vi "phasePlotWrap.vi"(6 "Sampling info":cluster{"Fs":dbl, "#s":dbl}={"Fs"=10000.0, "#s"=1000.0} {"Fs" format="%.2p"}, 8 "Phase unit":u16(ring) items=["Degree", "Radian"], 9 "Phase":dbl, 10 "Nomial Frequency":dbl, 11 "Frequency":dbl) -> (1 "yScaleMin":dbl, 2 "yScaleMax":dbl, 3 "Phase waveform":waveform(dbl)(graph))   [LabVIEW 2025]
uses:
  <vilib>/measure/NI_MAPro.lvlib
  <vilib>/measure/maresamp.llb/Align 1 + N Waveforms (continuous).vi
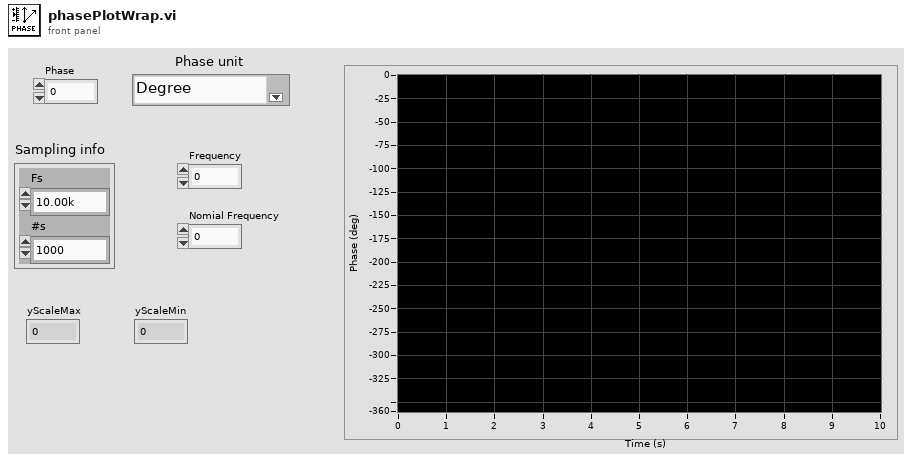
[diagram p1: front panel]
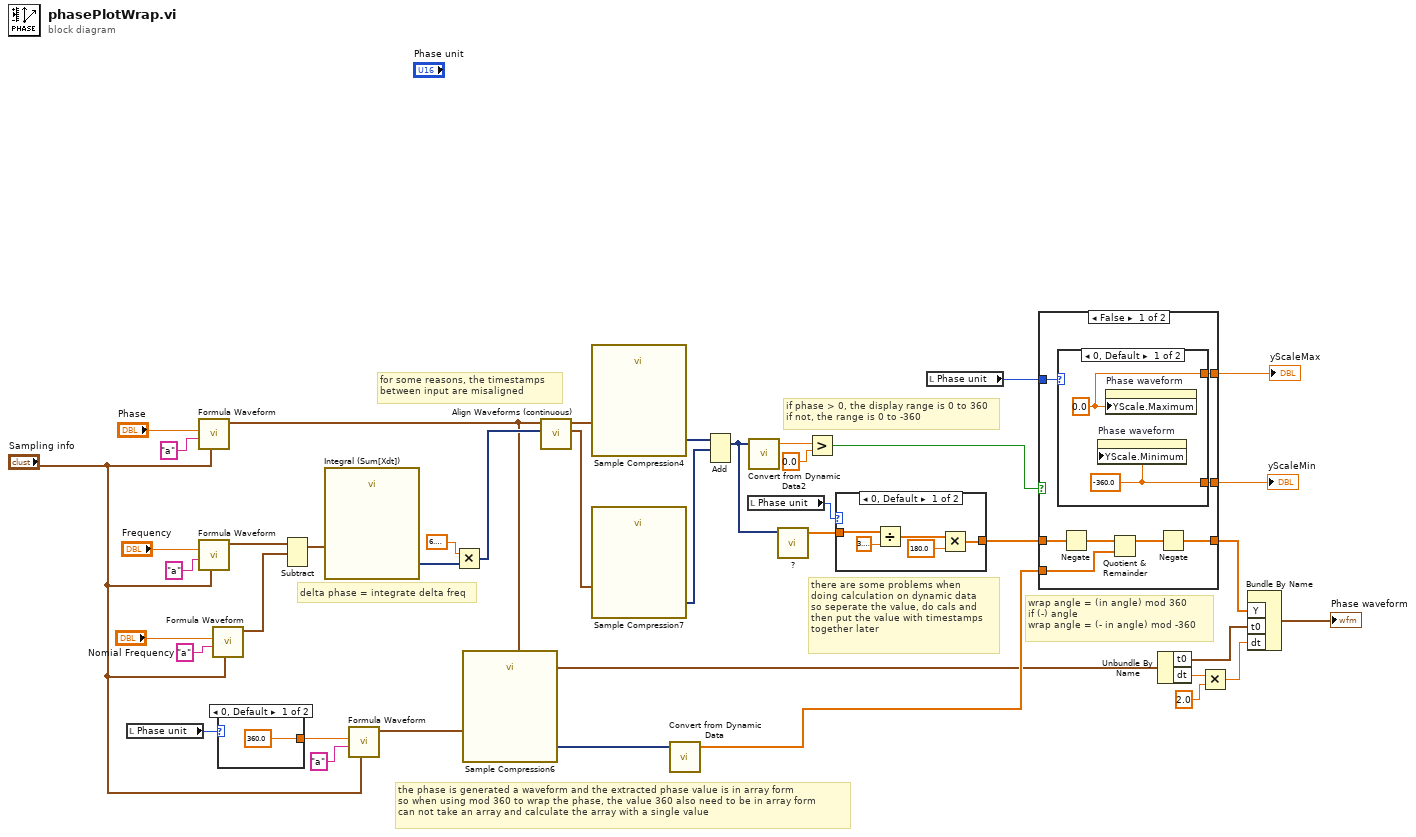
[diagram p0: block diagram]
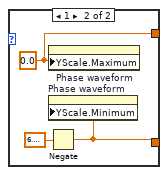
[diagram p2: hidden frame]
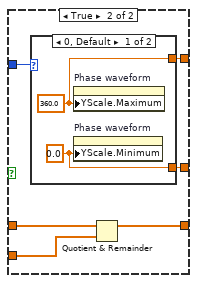
[diagram p3: hidden frame]
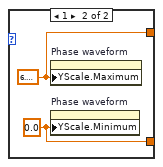
[diagram p4: hidden frame]
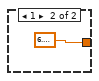
[diagram p6: hidden frame]
diagram:
  # "for some reasons, the timestamps \nbetween input are misaligned"
  # "there are some problems when\ndoing calculation on dynamic data\nso seperate the value, do cals and\nthen put the value with timestamps\ntogether later"
  # "wrap angle = (in angle) mod 360\nif (-) angle\nwrap angle = (- in angle) mod -360"
  # "if phase > 0, the display range is 0 to 360\nif not, the range is 0 to -360"
  # "the phase is generated a waveform and the extracted phase value is in array form\nso when using mod 360 to wrap the phase, the value 360 also need to be in array form\ncan not take an array and calculate the array with a single value"
  # "delta phase = integrate delta freq"
  n1 = local read "Phase unit"() -> (w31:u16)
  n2 = call <vilib>:"Formula Waveform.vi"("sampling info"="Sampling info", "formula"="a", "amplitude"="Phase") -> ("signal out"=w8:waveform(dbl))  [unwired: 7 in, 1 out]
  n3 = call <vilib>:"Formula Waveform.vi"("sampling info"="Sampling info", "formula"="a", "amplitude"="Frequency") -> ("signal out"=w33:waveform(dbl))  [unwired: 7 in, 1 out]
  n4 = call <vilib>:"Formula Waveform.vi"("sampling info"="Sampling info", "formula"="a", "amplitude"="Nomial Frequency") -> ("signal out"=w38:waveform(dbl))  [unwired: 7 in, 1 out]
  n5 = case shown="0, Default" w31 {
    tunnel: [360.0 6.283185307179586] -> w30
    frame 0, Default {
    }
    frame 1 {
    }
  }
  n6 = Subtract(1:w38, 2:w33) -> (0:w37:waveform(dbl))  [unwired: 1 in, 1 out]
  n7 = call "Integral (Sum[Xdt])"("Signals"=w37) -> ("Result"=w36:dynamicdata)  [unwired: 5 in, 1 out]
  n8 = call <vilib>:"Formula Waveform.vi"("sampling info"="Sampling info", "formula"="a", "amplitude"=w30) -> ("signal out"=w32:waveform(dbl))  [unwired: 7 in, 1 out]
  n9 = Multiply(x=6.283185307179586, y=w36) -> (x*y=w27:dynamicdata)
  n10 = call "Sample Compression6"("Signals"=w32) -> ("Maximum"=w29:dynamicdata)  [unwired: 8 in, 2 out]
  n11 = call-poly <vilib>:"Align Waveforms (continuous).vi"("waveforms in"=w27, "waveform in"=w8) -> ("aligned waveforms out"=w25:waveform(dbl)[], "aligned waveform out"=w26:waveform(dbl))  [unwired: 7 in, 1 out]
  n12 = call "Sample Compression4"("Signals"=w26) -> ("Maximum"=w24:dynamicdata)  [unwired: 8 in, 2 out]
  n13 = call "Sample Compression7"("Signals"=w25) -> ("Maximum"=w23:dynamicdata)  [unwired: 8 in, 2 out]
  n14 = call "Convert from Dynamic Data"("Dynamic Data Type"=w29) -> ("Array"=w9:dbl[])  [unwired: 3 in]
  n15 = Add(1:w23, 2:w24) -> (0:w10:dynamicdata)  [unwired: 1 in, 1 out]
  n16 = local read "Phase unit"() -> (w22:u16)
  n17 = call "Convert from Dynamic Data2"("Dynamic Data Type"=w10) -> ("Scalar"=w20:dbl)  [unwired: 3 in]
  n18 = call "?"("Dynamic Data Type"=w10) -> ("Array"=w21:dbl[])  [unwired: 3 in]
  n19 = Greater?(x=w20, y=0.0) -> (0:w19:bool)
  n20 = case shown="0, Default" w22 {
    tunnel: w21 -> [w44 w48]
    tunnel: [w43 w48] -> w17
    frame 0, Default {
      n21 = Divide(x=w44, y=3.141592653589793) -> (x/y=w47:dbl[])
      n22 = Multiply(x=w47, y=180.0) -> (x*y=w43:dbl[])
    }
    frame 1 {
    }
  }
  n23 = local read "Phase unit"() -> (w18:u16)
  n24 = case shown="False" w19 {
    tunnel: w18 -> [w56 w64]
    tunnel: w17 -> [w55 w67]
    tunnel: w9 -> [w53 w66]
    tunnel: [w51 w65] -> w13
    tunnel: [w50 w63] -> w5
    tunnel: [w49 w62] -> w4
    frame False {
      n25 = case shown="0, Default" w56 {
        tunnel: [w58 w60] -> w50
        tunnel: [w57 w59] -> w49
        frame 0, Default {
          w57 = -360.0 ("Y Scale.Range:Maximum")
          w58 = 0.0 ("Y Scale.Range:Maximum")
          n26 = property on="Phase waveform" class="WFChart (strict)"("YScale.Minimum"=w57) -> ()  [unwired: 2 in, 2 out]
          n27 = property on="Phase waveform" class="WFChart (strict)"("YScale.Maximum"=w58) -> ()  [unwired: 2 in, 2 out]
        }
        frame 1 {
          w60 = 0.0 ("Y Scale.Range:Minimum")
          n28 = Negate(x=6.283185307179586) -> (-x=w59:dbl)
          n29 = property on="Phase waveform" class="WFChart (strict)"("YScale.Maximum"=w60) -> ()  [unwired: 2 in, 2 out]
          n30 = property on="Phase waveform" class="WFChart (strict)"("YScale.Minimum"=w59) -> ()  [unwired: 2 in, 2 out]
        }
      }
      n31 = Negate(x=w55) -> (-x=w52:dbl[])
      n32 = Quotient & Remainder(x=w52, y=w53) -> (x-y*floor(x/y)=w54:dbl[])  [unwired: 1 out]
      n33 = Negate(x=w54) -> (-x=w51:dbl[])
    }
    frame True {
      n34 = case shown="0, Default" w64 {
        tunnel: [w69 w71] -> w63
        tunnel: [w68 w70] -> w62
        frame 0, Default {
          w68 = 0.0 ("Y Scale.Range:Maximum")
          w69 = 360.0 ("Y Scale.Range:Maximum")
          n35 = property on="Phase waveform" class="WFChart (strict)"("YScale.Maximum"=w69) -> ()  [unwired: 2 in, 2 out]
          n36 = property on="Phase waveform" class="WFChart (strict)"("YScale.Minimum"=w68) -> ()  [unwired: 2 in, 2 out]
        }
        frame 1 {
          w71 = 6.283185307179586
          w70 = 0.0 ("Y Scale.Range:Maximum")
          n37 = property on="Phase waveform" class="WFChart (strict)"("YScale.Maximum"=w71) -> ()  [unwired: 2 in, 2 out]
          n38 = property on="Phase waveform" class="WFChart (strict)"("YScale.Minimum"=w70) -> ()  [unwired: 2 in, 2 out]
        }
      }
      n39 = Quotient & Remainder(x=w67, y=w66) -> (x-y*floor(x/y)=w65:dbl[])  [unwired: 1 out]
    }
  }
  "yScaleMax" <- w5
  "yScaleMin" <- w4
  n40 = Unbundle By Name(w8) -> ("t0"=w15:timestamp, "dt"=w16:dbl)
  n41 = Multiply(x=w16, y=2.0) -> (x*y=w14:dbl)
  n42 = Bundle By Name("Y"=w13, "t0"=w15, "dt"=w14) -> (→"Phase waveform":waveform(dbl))  [unwired: 1 in]
